vi "IND560 Decode.vi"(8 "Error In":errorcluster, 11 "read buffer":string) -> (0 "Error Out":errorcluster, 2 "Displayed Net Wt.":dbl, 3 "Displayed Gross Wt.":dbl, 5 "Terminal Serial Number":string)   [LabVIEW 2014]
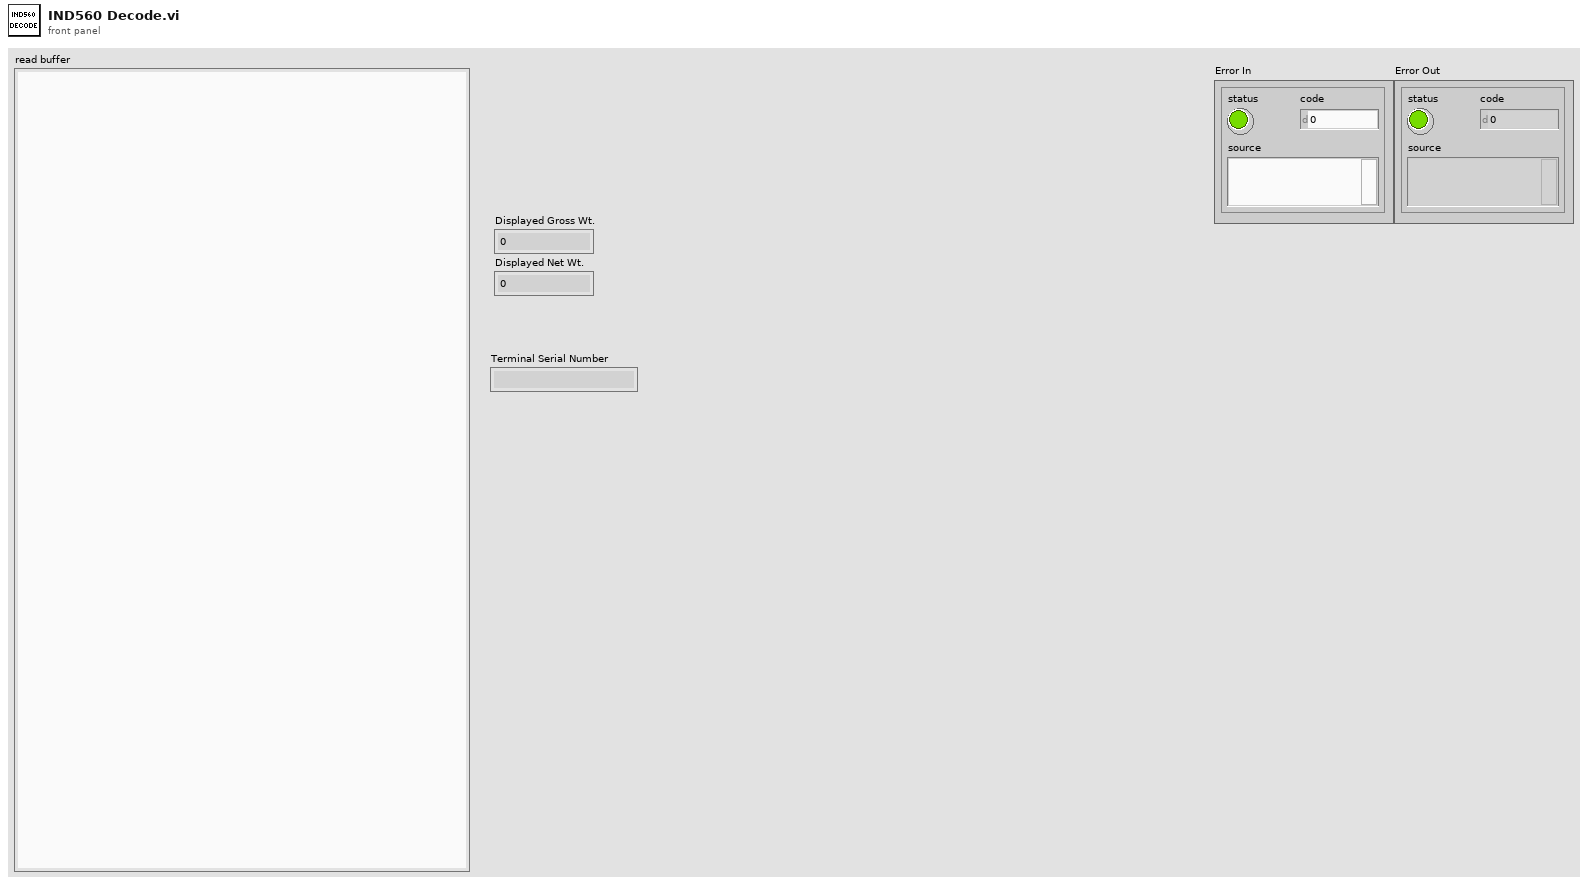
[diagram p1: front panel]
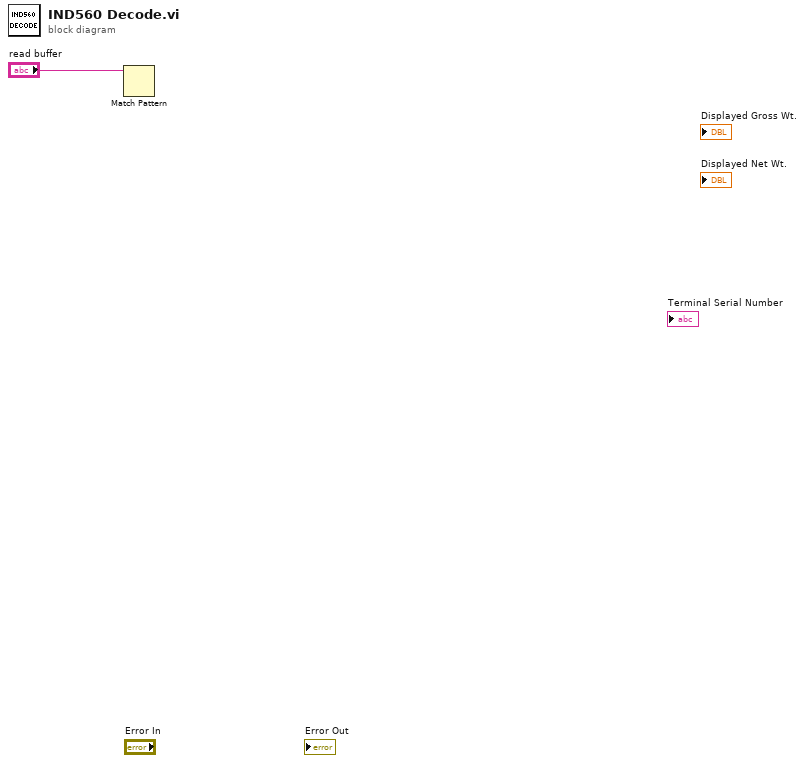
[diagram p0: block diagram]
diagram:
  n1 = Match Pattern(string="read buffer") -> ()  [unwired: 2 in, 4 out]
